vi "HeaderAction.vi"(0 "InstrClass":refnum<class "AttoAMC300.lvclass"> caption="DNL_LabVIEW Object in", 11 "error in (no error)":errorcluster caption="entrée d'erreur (pas d'erreur)") -> (4 "InstrClassOut":refnum<class "AttoAMC300.lvclass"> caption="DNL_LabVIEW Object out", 6 "DataNames":string[](array[string]), 8 "Instr Name":string, 10 "HeaderString":string, 13 "ArrDatNames":string[](array[string]), 14 "DisplayNames":string[](array[string]), 15 "error out":errorcluster caption="sortie d'erreur")   [LabVIEW 2019, in "AttoAMC300.lvclass"]
uses:
  AttoAMC300.lvclass
  C:/Programmes Labview/LabScanV1A/DevicesClass/BaseDevice/BaseDevice.lvclass
  AttoAMC300.lvclass/AttoAMC300.ctl
  <vilib>/Utility/error.llb/Error Cluster From Error Code.vi
  <vilib>/ErrorRing/Error Ring.xnode
  BaseDevice/BaseDevice.lvclass
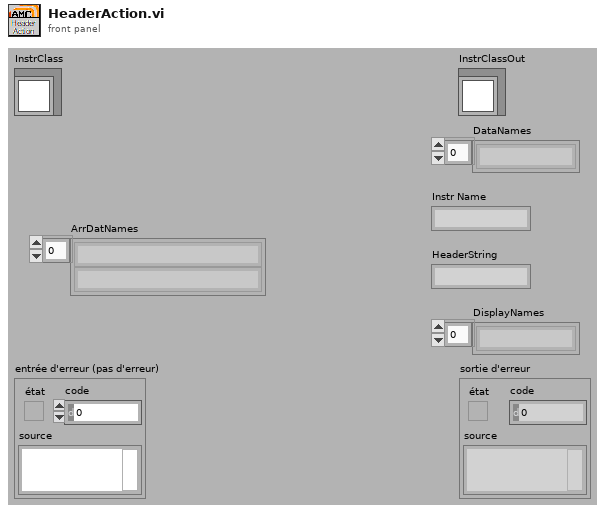
[diagram p1: front panel]
types:
  T1 = typedef "AttoAMC300.lvclass/AttoAMC300_Func.ctl" = enum16{"Position (um)", "MotionMon (um)"}
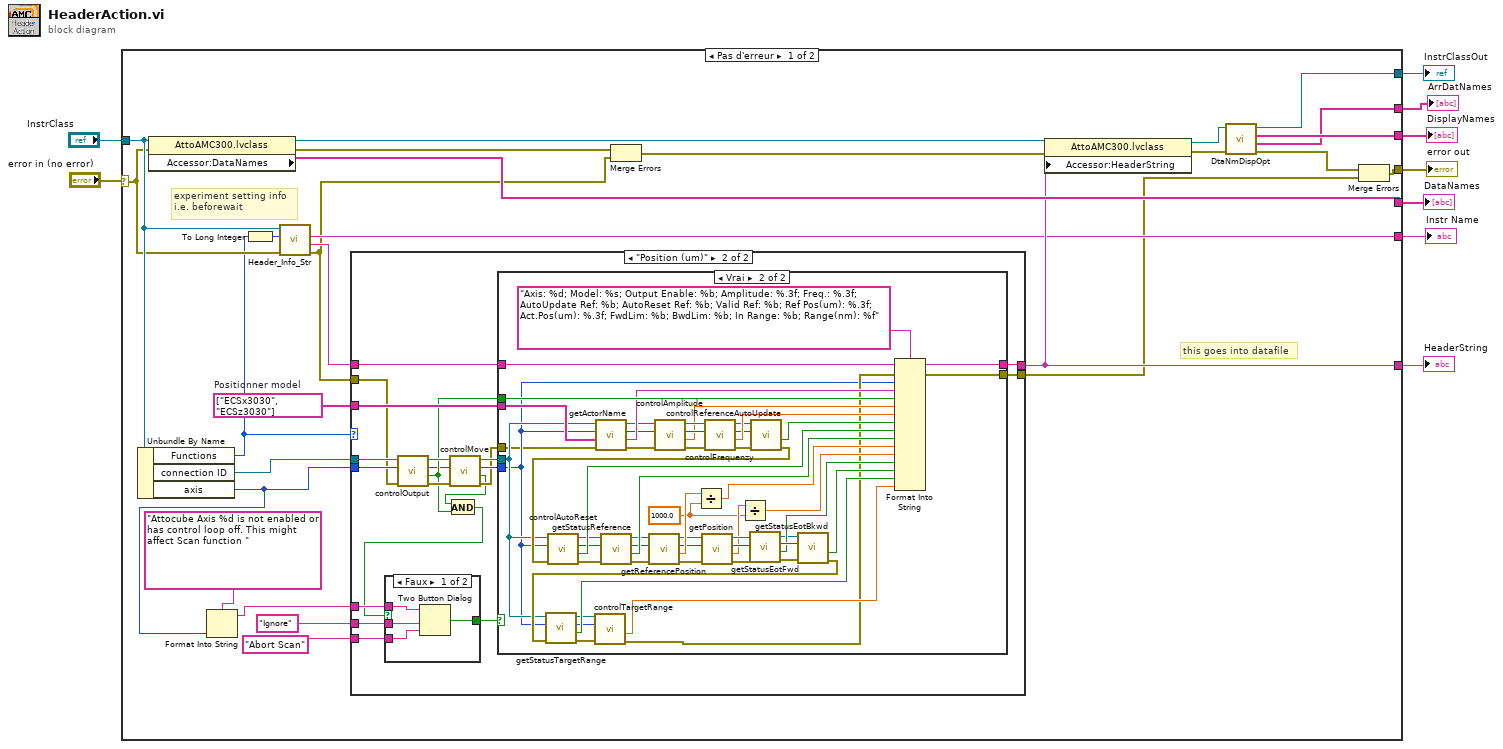
[diagram p0: block diagram]
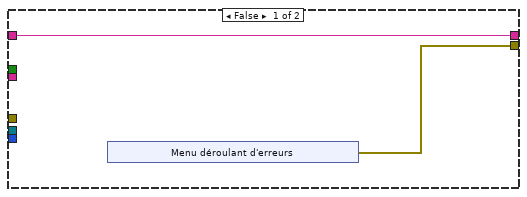
[diagram p4: hidden frame]
diagram:
  n1 = case shown="Pas d'erreur" "error in (no error)" {
    selector: "error in (no error)" -> [w26 w125]
    tunnel: [w33 _] -> w8
    tunnel: [w36 _] -> w7
    tunnel: "InstrClass" -> [w29 w126]
    tunnel: [w21 w125] -> w5
    tunnel: [w19 w126] -> w3
    tunnel: [w28 _] -> w4
    tunnel: [w30 _] -> w2
    tunnel: [w17 _] -> w1
    frame No Error {
      w22 = string[] ["ECSx3030", "ECSz3030"]  # Positionner model
      # "this goes into datafile"
      # "experiment setting info\ni.e. beforewait"
      n2 = Unbundle By Name(w29) -> ("Functions"=w24:T1, "connection ID"=w16:refnum<k5>, "axis"=w14:i32)
      n3 = property class="AttoAMC300.lvclass"(reference=w29, error in=w26) -> (reference out=w35:refnum<class "AttoAMC300.lvclass">, error out=w34:errorcluster, "Accessor:DataNames"=w36:string[])
      n4 = Format Into String(format string="Attocube Axis %d is not enabled or has control loop off. This might affect Scan function " ("message"), w14) -> (resulting string=w13:string)  [unwired: 2 in, 1 out]
      n5 = To Long Integer(number=w24) -> (32bit integer=w23:i32)
      n6 = call-dynamic "Header_Info_Str.vi"("error in (no error)"=w26, "Functions"=w23, "DefaultDev in"=w29) -> ("error out"=w10:errorcluster, "HdrInfoStr"=w27:string, "InstrumentName"=w28:string)  [unwired: 5 in, 1 out]
      n7 = case shown="\"Position (um)\"" w24 {
        tunnel: [w38 w56] -> w33
        tunnel: w27 -> [w38 w57]
        tunnel: w22 -> [_ w58]
        tunnel: w14 -> [_ w50]
        tunnel: w16 -> [_ w53]
        tunnel: w10 -> [w37 w49]
        tunnel: [w37 w55] -> w20
        tunnel: w13 -> [_ w43]
        tunnel: "Abort Scan" ("Nom du bouton F (\"Annuler\")") -> [_ w42]
        tunnel: "Ignore" ("Nom du bouton V (\"OK\")") -> [_ w41]
        frame Default {
        }
        frame "Position (um)" {
          n8 = call <userlib>:"controlOutput.vi"("error in"=w49, "axis in"=w50, "connection ID"=w53) -> ("error out"=w48:errorcluster, "enable output out"=w45:bool, "axis out"=w39:u8, "connection ID"=w54:refnum<k5>)  [unwired: 5 in]
          n9 = call <userlib>:"controlMove.vi"("error in"=w48, "axis in"=w39, "connection ID"=w54) -> ("error out"=w47:errorcluster, "controll move out"=w46:bool, "axis out"=w51:u8, "connection ID"=w52:refnum<k5>)  [unwired: 5 in]
          n10 = And(x=w46, y=w45) -> (x .and. y?=w40:bool)
          n11 = case shown="Faux" w40 {
            selector: w40 -> [_ w63]
            tunnel: [w62 w63] -> w44
            tunnel: w43 -> [w61 _]
            tunnel: w42 -> [w60 _]
            tunnel: w41 -> [w59 _]
            frame False {
              n12 = Two Button Dialog(message=w61, 1:w60, 2:w59) -> (T button?=w62:bool)
            }
            frame True {
            }
          }
          n13 = case shown="Vrai" w44 {
            tunnel: w58 -> [_ w124]
            tunnel: w57 -> [w65 w123]
            tunnel: w45 -> [_ w121]
            tunnel: [w65 w86] -> w56
            tunnel: [w64 w80] -> w55
            tunnel: w52 -> [_ w73]
            tunnel: w51 -> [_ w72]
            tunnel: w47 -> [_ w71]
            frame False {
              n14 = xnode "Menu déroulant d'erreurs"() -> ("sortie d'erreur"=w64:errorcluster)
            }
            frame True {
              w82 = 1000.0 ("y")
              n15 = call <userlib>:"getActorName.vi"("error in"=w71, "Actor Names"=w124, "axis in"=w72, "connection ID"=w73) -> ("error out"=w76:errorcluster, "ActorName out"=w78:string, "axis out"=w74:u8, "connection ID"=w75:refnum<k5>)  [unwired: 4 in]
              n16 = call <userlib>:"controlAmplitude.vi"("error in"=w76, "axis in"=w74, "connection ID"=w75) -> ("error out"=w118:errorcluster, "amplitude [V] out"=w117:dbl, "axis out"=w120:u8, "connection ID"=w119:refnum<k5>)  [unwired: 5 in]
              n17 = call <userlib>:"controlFrequenzy.vi"("error in"=w118, "axis in"=w120, "connection ID"=w119) -> ("error out"=w115:errorcluster, "Frequenzy [Hz] out"=w116:dbl, "axis out"=w113:u8, "connection ID"=w114:refnum<k5>)  [unwired: 5 in]
              n18 = call <userlib>:"controlReferenceAutoUpdate.vi"("error in"=w115, "axis in"=w113, "connection ID"=w114) -> ("error out"=w111:errorcluster, "ref auto up out"=w112:bool)  [unwired: 5 in, 2 out]
              n19 = call <userlib>:"controlAutoReset.vi"("error in"=w111, "axis in"=w72, "connection ID"=w73) -> ("error out"=w107:errorcluster, "auto reset out"=w110:bool, "axis out"=w108:u8, "connection ID"=w109:refnum<k5>)  [unwired: 5 in]
              n20 = call <userlib>:"getStatusReference.vi"("error in"=w107, "axis in"=w108, "connection ID"=w109) -> ("error out"=w103:errorcluster, "status reference out"=w106:bool, "axis out"=w101:u8, "connection ID"=w102:refnum<k5>)  [unwired: 5 in]
              n21 = call <userlib>:"getReferencePosition.vi"("error in"=w103, "axis in"=w101, "connection ID"=w102) -> ("error out"=w93:errorcluster, "Reference position out"=w105:dbl, "axis out"=w91:u8, "connection ID"=w92:refnum<k5>)  [unwired: 5 in]
              n22 = Divide(x=w105, y=w82) -> (x/y=w104:dbl)
              n23 = call <userlib>:"getPosition.vi"("error in"=w93, "axis in"=w91, "connection ID"=w92) -> ("error out"=w99:errorcluster, "position out"=w94:dbl, "axis out"=w98:u8, "connection ID"=w100:refnum<k5>)  [unwired: 5 in]
              n24 = Divide(x=w94, y=w82) -> (x/y=w90:dbl)
              n25 = call <userlib>:"getStatusEotFwd.vi"("error in"=w99, "axis in"=w98, "connection ID"=w100) -> ("error out"=w97:errorcluster, "Status EOT FWD out"=w89:bool, "axis out"=w95:u8, "connection ID"=w79:refnum<k5>)  [unwired: 5 in]
              n26 = call <userlib>:"getStatusEotBkwd.vi"("error in"=w97, "axis in"=w95, "connection ID"=w79) -> ("error out"=w96:errorcluster, "Get Stus EOT BKWD out"=w88:bool)  [unwired: 5 in, 2 out]
              n27 = call <userlib>:"getStatusTargetRange.vi"("error in"=w96, "axis in"=w72, "connection ID"=w73) -> ("error out"=w84:errorcluster, "Status Target Range out"=w87:bool, "axis out"=w83:u8, "connection ID"=w85:refnum<k5>)  [unwired: 5 in]
              n28 = call <userlib>:"controlTargetRange.vi"("error in"=w84, "axis in"=w83, "connection ID"=w85) -> ("error out"=w77:errorcluster, "Target Range out"=w81:dbl)  [unwired: 5 in, 2 out]
              n29 = Format Into String(format string="Axis: %d; Model: %s; Output Enable: %b; Amplitude: %.3f; Freq.: %.3f; AutoUpdate Ref: %b; AutoReset Ref: %b; Valid Ref: %b; Ref Pos(um): %.3f; Act.Pos(um): %.3f; FwdLim: %b; BwdLim: %b; In Range: %b; Range(nm): %f" ("chaîne de format"), initial string=w123, error in=w77, w72, w78, w121, w117, w116, w112, w110, w106, w104, w90, w89, w88, w87, w81) -> (resulting string=w86:string, error out=w80:errorcluster)
            }
          }
        }
      }
      n30 = Merge Errors(w34, w10) -> (w25:errorcluster)
      n31 = property class="AttoAMC300.lvclass"(reference=w35, error in=w25, "Accessor:HeaderString"=w33) -> (reference out=w31:refnum<class "AttoAMC300.lvclass">, error out=w32:errorcluster)
      n32 = call "DtaNmDispOpt.vi"("error in (no error)"=w32, "BaseDevice en entrée"=w31) -> ("error out"=w18:errorcluster, "ArrDisplayNames"=w17:string[], "DisplayNames"=w30:string[], "BaseDevice en sortie"=w19:refnum<class "AttoAMC300.lvclass">)  [unwired: 6 in]
      n33 = Merge Errors(w18, w20) -> (w21:errorcluster)
    }
    frame Error {
    }
  }
  "error out" <- w5
  "InstrClassOut" <- w3
  "DataNames" <- w7
  "HeaderString" <- w8
  "Instr Name" <- w4
  "DisplayNames" <- w2
  "ArrDatNames" <- w1
